vi "IMAQ-SaveContrast.vi"(1 "contraste":dbl, 2 "tiempo (ms)":u32, 3 "Grabar":refnum<vi>, 4 "Status":string) -> (0 "Archivo de texto":path)   [LabVIEW 2010]
uses:
  <vilib>/Utility/error.llb/DialogType.ctl
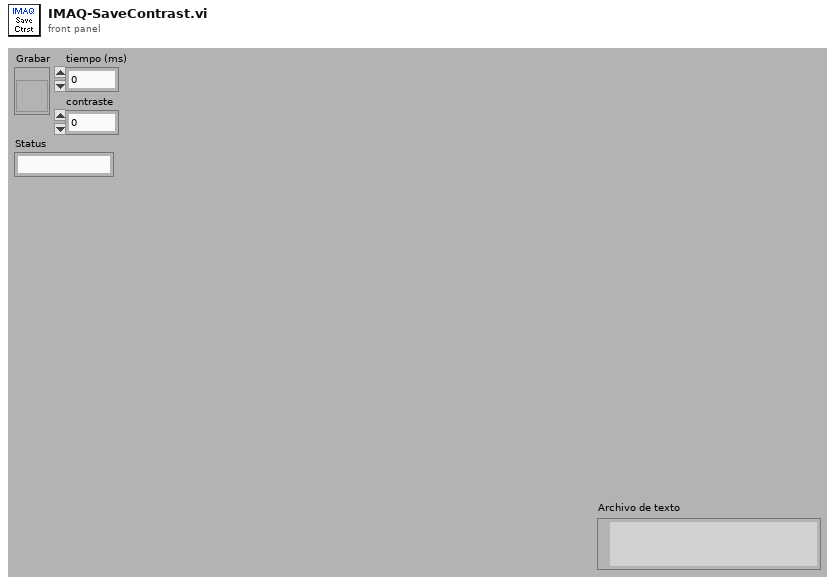
[diagram p1: front panel]
types:
  T1 = enum16{"open", "replace", "create", "open or create", "replace or create", "replace or create with confirmation"}
  T2 = enum32{"existing file", "new file", "new or existing file", "existing dir", "new dir", "new or existing dir", "existing file (use LLBs)", "new file (use LLBs)", "new or existing file (use LLBs)", "new or existing file or directory (use LLBs)"}
  T3 = typedef "DialogType.ctl" = u16
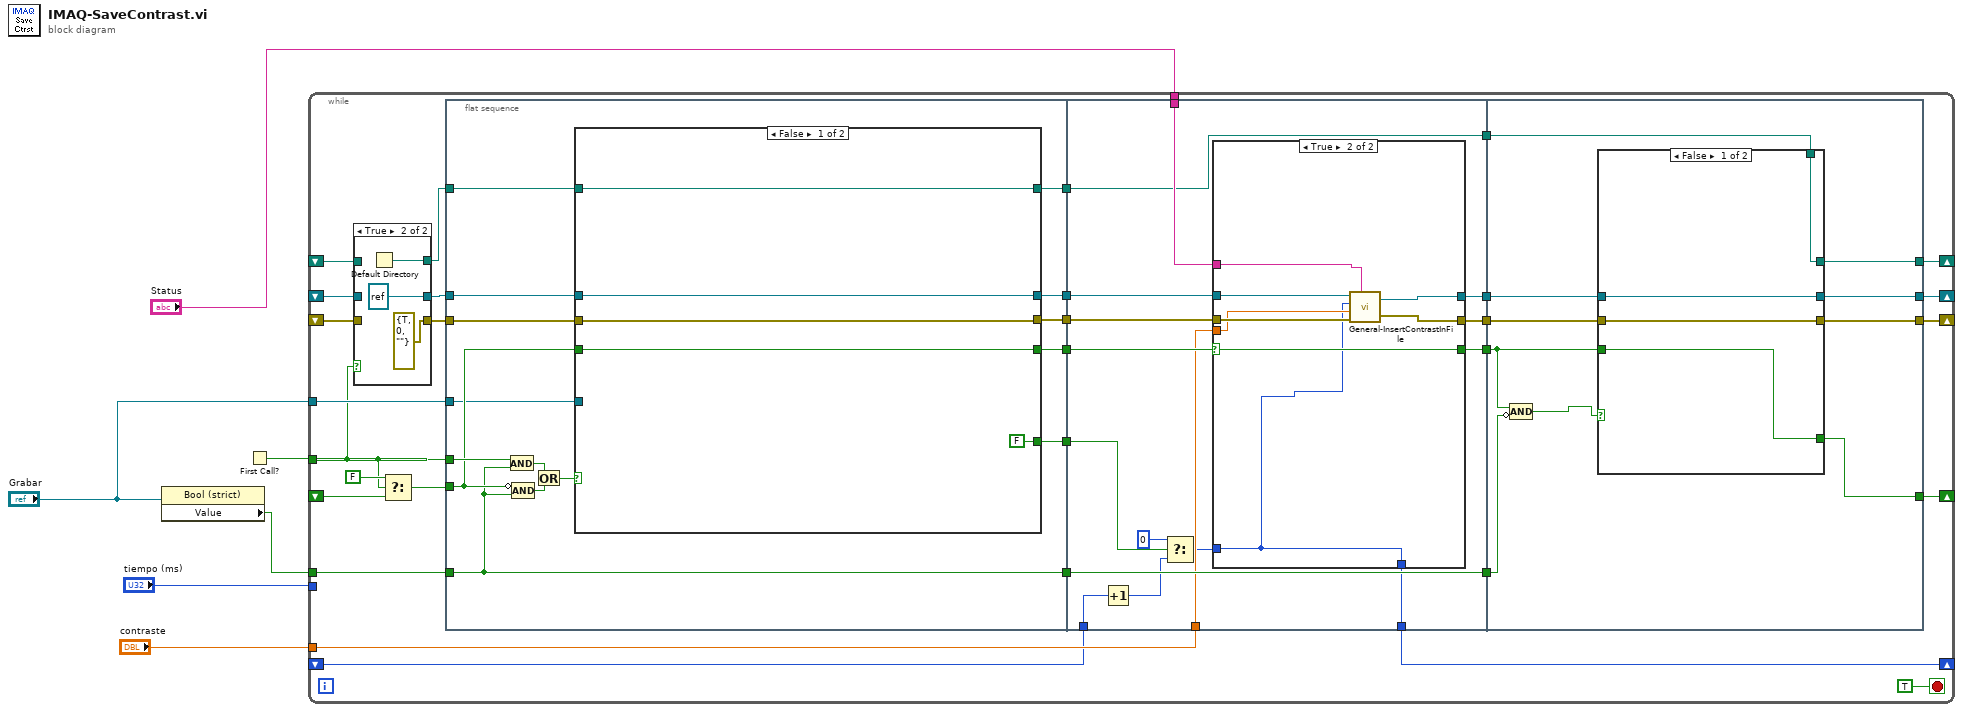
[diagram p0: block diagram]
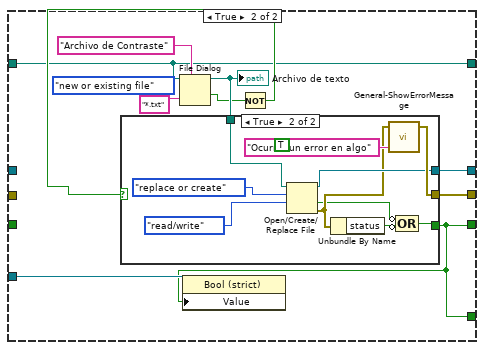
[diagram p3: hidden frame]
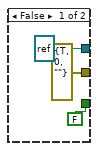
[diagram p4: hidden frame]
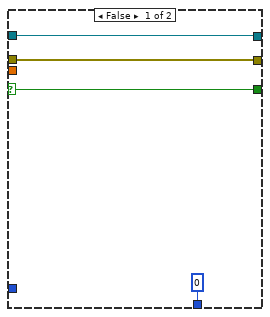
[diagram p5: hidden frame]
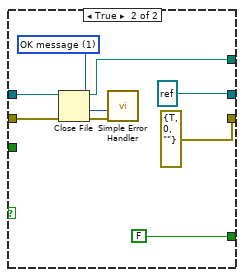
[diagram p6: hidden frame]
diagram:
  n1 = property class="Bool (strict)"(reference="Grabar") -> ("Value"=w5:bool)  [unwired: 1 in, 2 out]
  n2 = First Call?() -> (First Call?: T/F=w6:bool)
  n3 = while {
    tunnel: w6 -> [w13]
    tunnel: w5 -> [w37]
    shift-right: [w23] -> _
    shift-left: _ -> [w35]
    shift-right: [w28] -> _
    shift-left: _ -> [w21]
    shift-right: [w27] -> _
    shift-left: _ -> [w19]
    tunnel: "Grabar" -> [w18]
    tunnel: "tiempo (ms)" -> [_]
    tunnel: "contraste" -> [w17]
    shift-right: [w16] -> _
    shift-left: _ -> [w14]
    tunnel: "Status" -> [w12]
    shift-right: [w11] -> _
    shift-left: _ -> [w10]
    stop <- TRUE stop-if-true
    n4 = case shown="True" w13 {
      tunnel: [w41 refnum<file> refnum ("refnum OUT")] -> w22
      tunnel: w21 -> [w41 _]
      tunnel: [w40 errorcluster {"status"=TRUE, "code"=0, "source"=""} ("error out")] -> w20
      tunnel: w19 -> [w40 _]
      tunnel: w10 -> [w39 _]
      tunnel: [w39 w42] -> w9
      frame False {
      }
      frame True {
        n5 = Default Directory() -> (w42:path)
      }
    }
    n6 = Select(t=FALSE, s=w13, f=w35) -> (s? t:f=w34:bool)
    n7 = flat-sequence {
      tunnel: w13 -> [w56]
      tunnel: w37 -> [w49]
      tunnel: w34 -> [w52]
      tunnel: [w55] -> w33
      tunnel: [w54] -> w32
      tunnel: [w53] -> w31
      tunnel: w22 -> [w51]
      tunnel: w20 -> [w50]
      tunnel: [w49] -> w26
      tunnel: w18 -> [w48]
      tunnel: [w47] -> w15
      tunnel: w9 -> [w46]
      tunnel: [w45] -> w8
      tunnel: w33 -> [w103]
      tunnel: w32 -> [w96]
      tunnel: w31 -> [w102]
      tunnel: [w101] -> w30
      tunnel: [w100] -> w29
      tunnel: w26 -> [w99]
      tunnel: [w99] -> w25
      tunnel: [w98] -> w24
      tunnel: w17 -> [w97]
      tunnel: [w95] -> w16
      tunnel: w15 -> [w94]
      tunnel: w14 -> [w90]
      tunnel: w12 -> [w89]
      tunnel: w8 -> [w88]
      tunnel: [w88] -> w7
      tunnel: w30 -> [w125]
      tunnel: w29 -> [w124]
      tunnel: [w123] -> w28
      tunnel: [w122] -> w27
      tunnel: w25 -> [w121]
      tunnel: w24 -> [w119]
      tunnel: [w120] -> w23
      tunnel: [w117] -> w11
      tunnel: w7 -> [w116]
      frame #0 {
        n8 = And(x=w56, y=w49) -> (x .and. y?=w58:bool)
        n9 = Compound Arithmetic op=AND(invert w52, w49) -> (w57:bool)
        n10 = Or(x=w58, y=w57) -> (x .or. y?=w59:bool)
        n11 = case shown="False" w59 {
          tunnel: [w63 w73] -> w55
          tunnel: [w62 w72] -> w54
          tunnel: [w64 w66] -> w53
          tunnel: w52 -> [w64 _]
          tunnel: w51 -> [w62 _]
          tunnel: w50 -> [w63 _]
          tunnel: w48 -> [_ w74]
          tunnel: [FALSE w66] -> w47
          tunnel: w46 -> [w60 w65]
          tunnel: [w60 w65] -> w45
          frame False {
          }
          frame True {
            (unwired) T2."new or existing file" ("select mode (2)")
            n12 = File Dialog(6:"*.txt" ("pattern"), 7:"Archivo de Contraste" ("prompt"), 11:w65) -> (1:w68:bool, 3:w69:path)  [unwired: 1 in, 5 out]
            "Archivo de texto" <- w69
            n13 = Not(x=w68) -> (.not. x?=w67:bool)
            n14 = case shown="True" w67 {
              tunnel: [errorcluster {"status"=TRUE, "code"=0, "source"=""} ("Error OUT") w87] -> w73
              tunnel: w69 -> [_ w85]
              tunnel: [refnum<file> refnum ("refnum out") w82] -> w72
              tunnel: [FALSE w78] -> w66
              frame False {
              }
              frame True {
                (unwired) TRUE ("Has Data")
                n15 = Open/Create/Replace File(file path (use dialog)=w85, operation (0:open)=T1."replace or create", access (0:read/write)=enum16{"read/write", "read-only", "write-only"}."read/write") -> (refnum out=w82:refnum<file>, cancelled=w79:bool, error out=w81:errorcluster)  [unwired: 3 in]
                n16 = Unbundle By Name(w81) -> ("status"=w80:bool)
                n17 = call "General-ShowErrorMessage.vi"("message"="Ocurrio un error en algo", "Error IN"=w81) -> ("Error OUT"=w87:errorcluster)  [unwired: 3 in]
                n18 = Compound Arithmetic op=OR(invert w79, invert w80) -> (w78:bool)
              }
            }
            n19 = property class="Bool (strict)"(reference=w74, "Value"=w66) -> ()  [unwired: 1 in, 2 out]
          }
        }
      }
      frame #1 {
        n20 = Increment(x=w90) -> (x+1=w91:u32)
        n21 = Select(t=u32 0, s=w94, f=w91) -> (s? t:f=w93:u32)
        n22 = case shown="True" w102 {
          selector: w102 -> [w106 w115]
          tunnel: w103 -> [w107 w114]
          tunnel: w96 -> [w105 w110]
          tunnel: [w107 w113] -> w101
          tunnel: [w105 w111] -> w100
          tunnel: [w106 w115] -> w98
          tunnel: w97 -> [_ w112]
          tunnel: w93 -> [_ w109]
          tunnel: [u32 0 ("t") w109] -> w95
          tunnel: w89 -> [_ w108]
          frame False {
          }
          frame True {
            n23 = call "General-InsertContrastInFile.vi"("refnum IN"=w110, "tiempo (ms)"=w109, "contraste"=w112, "error IN"=w114, "Status"=w108) -> ("refnum OUT"=w111:refnum<file>, "error OUT"=w113:errorcluster)
          }
        }
      }
      frame #2 {
        n24 = Compound Arithmetic op=AND(w119, invert w121) -> (w118:bool)
        n25 = case shown="False" w118 {
          tunnel: w125 -> [w128 w136]
          tunnel: w124 -> [w129 w132]
          tunnel: [w129 refnum<file> refnum ("refnum OUT")] -> w123
          tunnel: [w128 errorcluster {"status"=TRUE, "code"=0, "source"=""} ("error out")] -> w122
          tunnel: [w127 FALSE] -> w120
          tunnel: w119 -> [w127 _]
          tunnel: [w126 w130] -> w117
          tunnel: w116 -> [w126 _]
          frame False {
          }
          frame True {
            w133 = T3 1 items=["no dialog", "OK message", "continue or stop message", "OK message + warnings", "continue/stop + warnings"] ("type of dialog (OK msg:1)")
            n26 = Close File(refnum=w132, error in=w136) -> (path=w130:path, error out=w137:errorcluster)
            n27 = call <vilib>:"Simple Error Handler.vi"("type of dialog (OK msg:1)"=w133, "error in (no error)"=w137) -> ()  [unwired: 8 out]
          }
        }
      }
    }
  }
